vi "Get Full Data.vi"(8 "error in (no error)":errorcluster, 11 "nmea in":refnum<class "nmea.lvclass">) -> (0 "error out":errorcluster, 2 "Full Data":T1 {"Fix"."Longitude" format="%_16f"; "Fix"."Latitude" format="%_16f"}, 3 "nmea out":refnum<class "nmea.lvclass">)   [LabVIEW 2012, in "nmea.lvlib" / "nmea.lvclass"]
uses:
  nmea.lvclass
  Fix.ctl
  Velocity.ctl
  DOP.ctl
  Satellite.ctl
  Fix Type.ctl
  Fix Mode.ctl
  Full Data.ctl
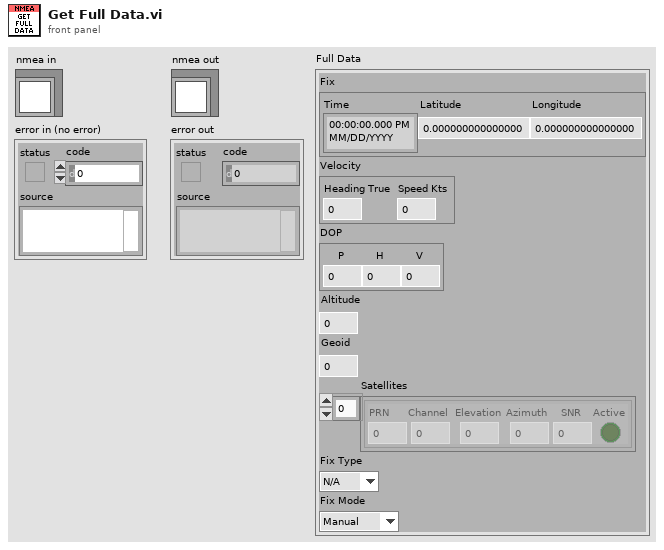
[diagram p1: front panel]
types:
  T1 = typedef "nmea.lvlib/nmea.lvclass/Full Data.ctl" = cluster{"Fix":T2, "Velocity":T3, "DOP":T4, "Altitude":dbl, "Geoid":dbl, "Satellites":T5[], "Fix Type":T6, "Fix Mode":T7}
  T2 = typedef "nmea.lvlib/nmea.lvclass/Fix.ctl" = cluster{"Time":timestamp, "Latitude":dbl, "Longitude":dbl}
  T3 = typedef "nmea.lvlib/nmea.lvclass/Velocity.ctl" = cluster{"Heading True":dbl, "Speed Kts":dbl}
  T4 = typedef "nmea.lvlib/nmea.lvclass/DOP.ctl" = cluster{"P":dbl, "H":dbl, "V":dbl}
  T5 = typedef "nmea.lvlib/nmea.lvclass/Satellite.ctl" = cluster{"PRN":u8, "Channel":u8, "Elevation":u8, "Azimuth":u16, "SNR":u8, "Active":bool}
  T6 = typedef "nmea.lvlib/nmea.lvclass/Fix Type.ctl" = enum16{"N/A", "None", "2D", "3D"}
  T7 = typedef "nmea.lvlib/nmea.lvclass/Fix Mode.ctl" = enum16{"Manual", "Auto 2/3D"}
  T8 = typedef "nmea.lvlib/nmea.lvclass/Ref Data.ctl" = cluster{"Latitude":dbl, "Longitude":dbl, "Time":T9, "Status":string, "Speed":dbl, "Course":dbl, "Mag Var":dbl, "Var Dir":string, "Mode":string, "Satellites":T5[], "Next Satellites":T5[], "Active PRNs":i32[], "Fix Type":T6, "DOP":T4, "Fix Mode":T7, "Altitude":dbl, "Geoid":dbl}
  T9 = typedef "LVDateTimeRec.ctl" = cluster{"fractional second":dbl, "second":i32, "minute":i32, "hour":i32, "day of month":i32, "month":i32, "year":i32, "day of week":i32, "day of year":i32, "DST":i32}
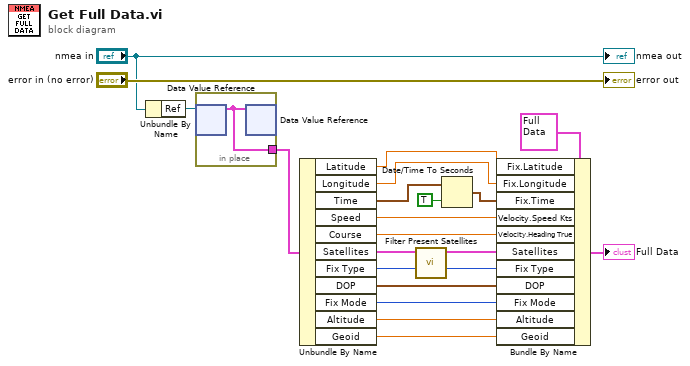
[diagram p0: block diagram]
diagram:
  n1 = Unbundle By Name("nmea in") -> ("Ref"=w19:refnum<data-value>)
  n2 = in-place {
    in-place-border: [w21] -> w15
    n3 = in-place-dvr #1(w19) -> (w21:T8)  [unwired: 1 out]
    n4 = in-place-dvr #1(w21) -> ()  [unwired: 2 out]
  }
  n5 = Unbundle By Name(w15) -> ("Latitude"=w10:dbl, "Longitude"=w9:dbl, "Time"=w14:T9, "Speed"=w11:dbl, "Course"=w8:dbl, "Satellites"=w2:T5[], "Fix Type"=w7:T6, "DOP"=w6:T4, "Fix Mode"=w5:T7, "Altitude"=w4:dbl, "Geoid"=w3:dbl)
  n6 = call "Filter Present Satellites.vi"("Satellites"=w2) -> ("Filtered Satellites"=w1:T5[])  [unwired: 10 in]
  n7 = Date/Time To Seconds(1:TRUE ("is UTC (F)"), 2:w14) -> (0:w12:timestamp)
  n8 = Bundle By Name(cluster=T1 {"Fix"={"Time"=timestamp(0 s since 1904-01-01), "Latitude"=0.0, "Longitude"=0.0}, "Velocity"={"Heading True"=0.0, "Speed Kts"=0.0}, "DOP"={"P"=0.0, "H"=0.0, "V"=0.0}, "Altitude"=0.0, "Geoid"=0.0, "Satellites"=[], "Fix Type"=enum."N/A", "Fix Mode"=enum."Manual"} ("Full Data"), "Fix.Latitude"=w10, "Fix.Longitude"=w9, "Fix.Time"=w12, "Velocity.Speed Kts"=w11, "Velocity.Heading True"=w8, "Satellites"=w1, "Fix Type"=w7, "DOP"=w6, "Fix Mode"=w5, "Altitude"=w4, "Geoid"=w3) -> (→"Full Data":T1)
  "error out" <- "error in (no error)"
  "nmea out" <- "nmea in"
